vi "Read Index Rect.vi"(9 "Array in":refnum<class "Array.lvclass">) -> (3 "Array out":refnum<class "Array.lvclass">, 4 "Index Rect":T1)   [LabVIEW 2014, in "Array.lvclass"]
uses:
  Array.lvclass
  <vilib>/Utility/miscctls.llb/LVRectTypeDef.ctl
  Array.lvclass/Array.ctl
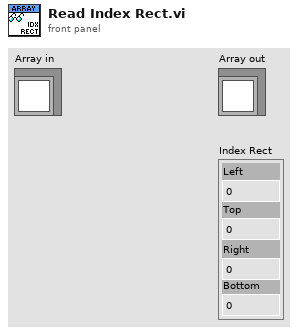
[diagram p1: front panel]
types:
  T1 = typedef "LVRectTypeDef.ctl" = cluster{"Left":i16, "Top":i16, "Right":i16, "Bottom":i16}
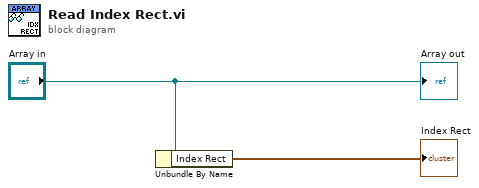
[diagram p0: block diagram]
diagram:
  n1 = Unbundle By Name("Array in") -> ("Index Rect"=→"Index Rect":T1)
  "Array out" <- "Array in"
